vi "Use Case2.vi"() -> ()   [LabVIEW 2021, in "uCanDriver.lvlib" / "uCAN.lvclass"]
uses:
  uCAN.lvclass
  typedefs/frame.ctl
  typedefs/bitrates.ctl
panel:
  in  "New Frame":T1 {"Data" format="%.0x"}
  in  "Bitrates":T2=enum."500 kbit/s"
  in  "COM port":refnum<visa-resource-name>="COM9"
  in  "Transmit Frame":bool
  in  "stop":bool
  out "Received Frames":T1[](array[typedef]) {"Data" format="%.0x"}
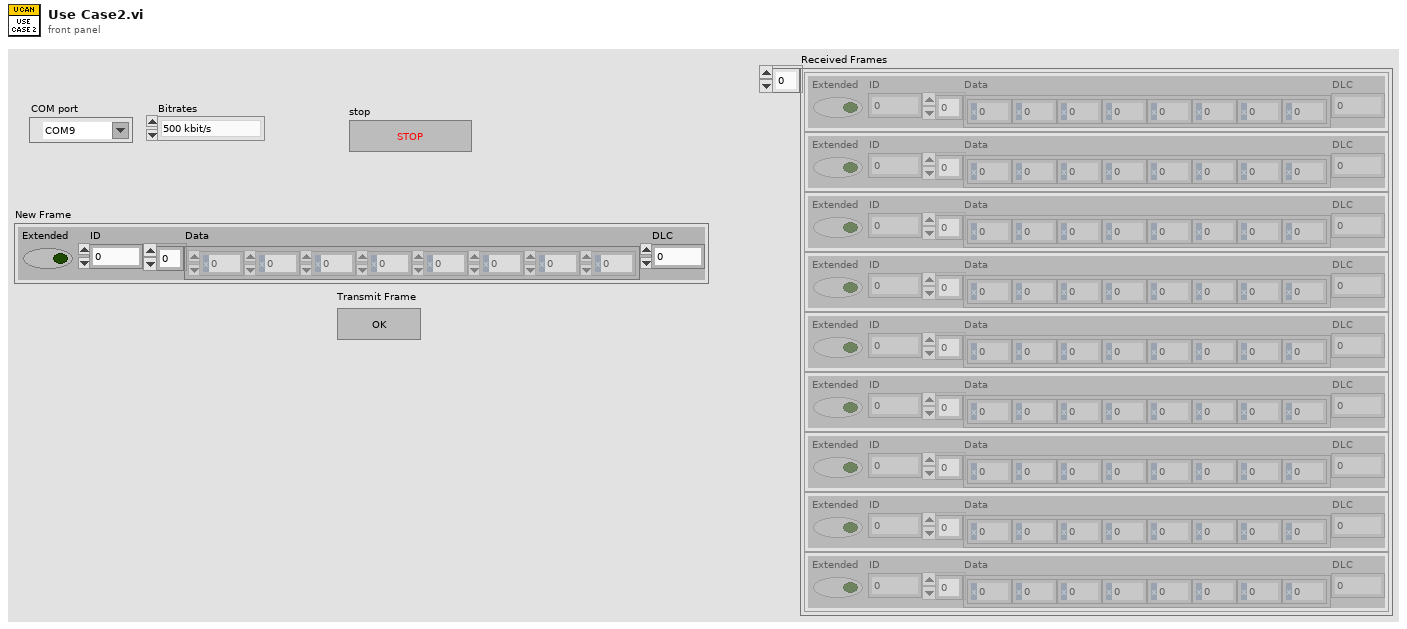
[diagram p1: front panel]
types:
  T1 = typedef "uCanDriver.lvlib/uCAN.lvclass/frame.ctl" = cluster{"Extended":bool, "ID":u32, "Data":u8[], "DLC":u8}
  T2 = typedef "uCanDriver.lvlib/uCAN.lvclass/bitrates.ctl" = enum16{"100 kbit/s", "125 kbit/s", "250 kbit/s", "500 kbit/s", "800 kbit/s", "1 Mbit/s"}
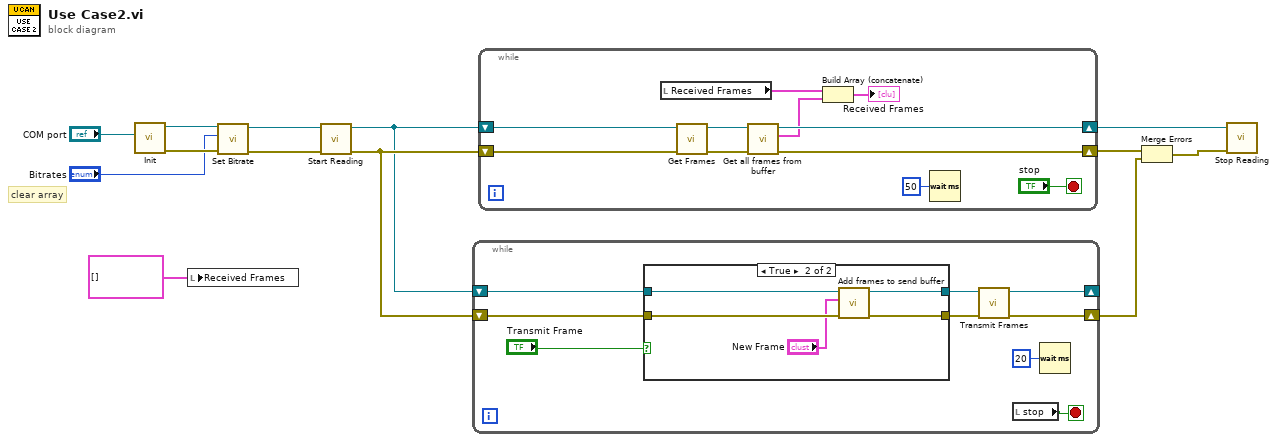
[diagram p0: block diagram]
diagram:
  # "clear array"
  n1 = call "Init.vi"("COM port"="COM port") -> ("error out"=w11:errorcluster, "uCAN out"=w12:refnum<class "uCAN.lvclass">)  [unwired: 9 in]
  n2 = local write "Received Frames"(T1[] [] ("Received Frames Array")) -> ()
  n3 = call "Set Bitrate.vi"("error in (no error)"=w11, "Bitrates"="Bitrates", "uCAN in"=w12) -> ("error out"=w4:errorcluster, "uCAN out"=w2:refnum<class "uCAN.lvclass">)  [unwired: 7 in]
  n4 = call "Start Reading.vi"("error in (no error)"=w4, "uCAN in"=w2) -> ("error out"=w3:errorcluster, "uCAN out"=w1:refnum<class "uCAN.lvclass">)  [unwired: 8 in]
  n5 = while {
    shift-right: [w16] -> _
    shift-left: w1 -> [w22]
    shift-right: [w18] -> w5
    shift-left: w3 -> [w21]
    stop <- w15 stop-if-true
    n6 = case shown="True" "Transmit Frame" {
      tunnel: w22 -> [w24 w29]
      tunnel: w21 -> [w23 w28]
      tunnel: [w23 w27] -> w20
      tunnel: [w24 w26] -> w17
      frame False {
      }
      frame True {
        n7 = call "Add frames to send buffer.vi"("error in (no error)"=w28, "New Frame"="New Frame", "uCAN in"=w29) -> ("error out"=w27:errorcluster, "uCAN out"=w26:refnum<class "uCAN.lvclass">)  [unwired: 7 in]
      }
    }
    n8 = call "Transmit Frames.vi"("error in (no error)"=w20, "uCAN in"=w17) -> ("error out"=w18:errorcluster, "uCAN out"=w16:refnum<class "uCAN.lvclass">)  [unwired: 8 in]
    n9 = local read "stop"() -> (w15:bool)
    n10 = Wait (ms)(milliseconds to wait=u32 20) -> ()  [unwired: 1 out]
  }
  n11 = while {
    shift-right: [w36] -> w9
    shift-left: w1 -> [w40]
    shift-right: [w35] -> w8
    shift-left: w3 -> [w39]
    stop <- "stop" stop-if-true
    n12 = local read "Received Frames"() -> (w31:T1[])
    n13 = call "Get Frames.vi"("error in (no error)"=w39, "uCAN in"=w40) -> ("error out"=w38:errorcluster, "uCAN out"=w37:refnum<class "uCAN.lvclass">)  [unwired: 7 in, 1 out]
    n14 = call "Get all frames from buffer.vi"("error in (no error)"=w38, "uCAN in"=w37) -> ("error out"=w35:errorcluster, "Received Frames Array"=w30:T1[], "uCAN out"=w36:refnum<class "uCAN.lvclass">)  [unwired: 7 in]
    n15 = Build Array (concatenate)(w31, w30) -> (→"Received Frames":T1[])
    n16 = Wait (ms)(milliseconds to wait=u32 50) -> ()  [unwired: 1 out]
  }
  n17 = Merge Errors(w8, w5) -> (w6:errorcluster)
  n18 = call "Stop Reading.vi"("error in (no error)"=w6, "uCAN in"=w9) -> ()  [unwired: 8 in, 2 out]
